vi "20220107_00.vi"() -> ()   [LabVIEW 2019]
uses:
  <vilib>/numeric/Random Number (Range) DBL.vi
panel:
  in  "Flush":bool
  out "enque timed out?":bool
  out "deque timed out?":bool
  out "element":dbl
  in  "Deque":bool
  out "elements":dbl[](array[numeric])
  in  "Lossy Enque":bool
  in  "Enque":bool
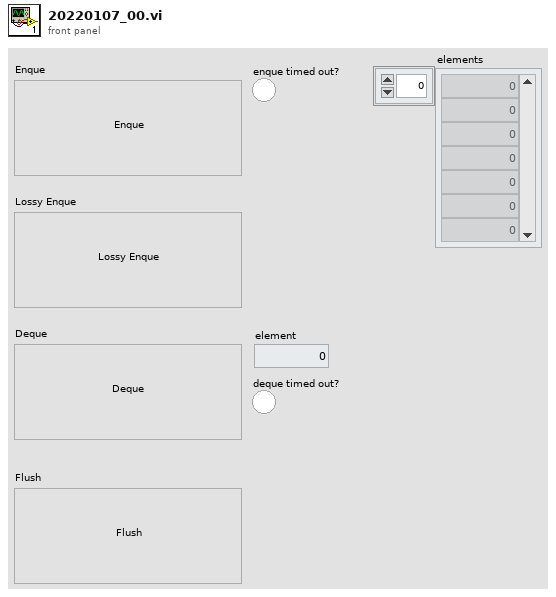
[diagram p1: front panel]
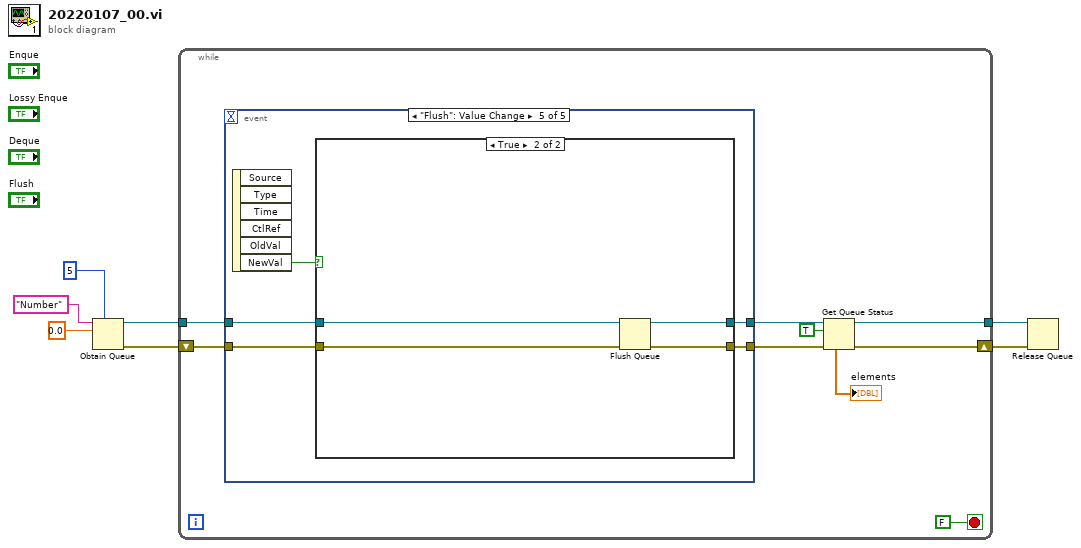
[diagram p0: block diagram]
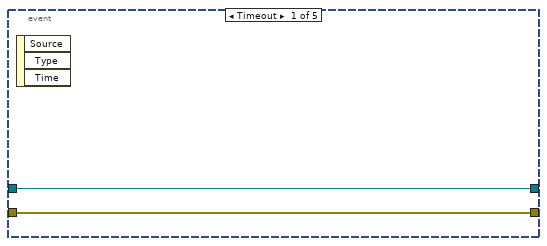
[diagram p2: hidden frame]
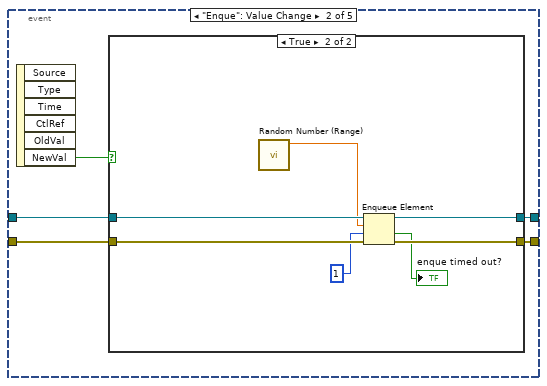
[diagram p3: hidden frame]
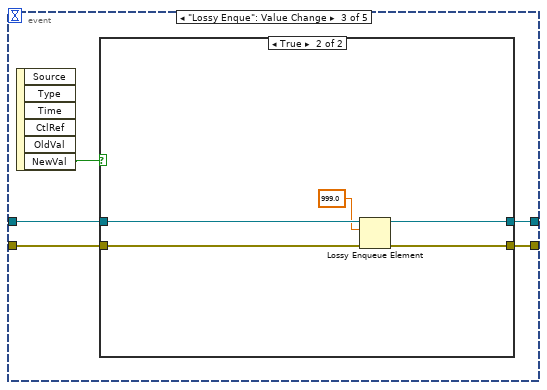
[diagram p5: hidden frame]
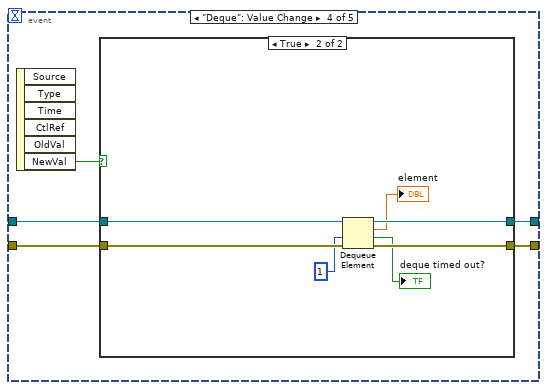
[diagram p7: hidden frame]
diagram:
  n1 = Obtain Queue(max queue size (-1, unlimited)=5, name (unnamed)="Number", element data type=0.0) -> (queue out=w2:refnum<queue>, error out=w3:errorcluster)  [unwired: 2 in, 1 out]
  n2 = while {
    shift-right: [w11] -> w5
    shift-left: w3 -> [w15]
    tunnel: w2 -> [w16]
    tunnel: [w10] -> w4
    stop <- FALSE stop-if-true
    n3 = event shown="[4] \"Flush\": Value Change" {
      selector: _ -> [_ _ _ _ _]
      dyn-events: _ -> [_ _ _ _ _]
      timeout: _ -> [_ _ _ _ _]
      tunnel: w16 -> [w17 w22 w35 w47 w61]
      tunnel: w15 -> [w18 w21 w36 w48 w62]
      tunnel: [w18 w20 w34 w46 w60] -> w13
      tunnel: [w17 w19 w33 w45 w59] -> w12
      event Timeout {
        n4 = event-data() -> ()  [unwired: 1 in, 3 out]
      }
      event "Enque": Value Change {
        n5 = event-data() -> ("NewVal"=w23:bool)  [unwired: 1 in, 5 out]
        n6 = case shown="True" w23 {
          tunnel: w22 -> [w24 w32]
          tunnel: w21 -> [w25 w31]
          tunnel: [w25 w30] -> w20
          tunnel: [w24 w29] -> w19
          frame False {
          }
          frame True {
            n7 = call-poly <vilib>:"Random Number (Range).vi"() -> ("number"=w28:dbl)  [unwired: 11 in]
            n8 = Enqueue Element(queue=w32, element=w28, timeout in ms (-1)=1, error in (no error)=w31) -> (queue out=w29:refnum<queue>, timed out?=→"enque timed out?":bool, error out=w30:errorcluster)
          }
        }
      }
      event "Lossy Enque": Value Change {
        n9 = event-data() -> ("NewVal"=w37:bool)  [unwired: 1 in, 5 out]
        n10 = case shown="True" w37 {
          tunnel: w36 -> [w39 w44]
          tunnel: w35 -> [w38 w43]
          tunnel: [w39 w42] -> w34
          tunnel: [w38 w41] -> w33
          frame False {
          }
          frame True {
            n11 = Lossy Enqueue Element(queue=w43, element=999.0, error in (no error)=w44) -> (queue out=w41:refnum<queue>, error out=w42:errorcluster)  [unwired: 2 out]
          }
        }
      }
      event "Deque": Value Change {
        n12 = event-data() -> ("NewVal"=w49:bool)  [unwired: 1 in, 5 out]
        n13 = case shown="True" w49 {
          tunnel: w48 -> [w51 w58]
          tunnel: w47 -> [w50 w57]
          tunnel: [w51 w56] -> w46
          tunnel: [w50 w55] -> w45
          frame False {
          }
          frame True {
            n14 = Dequeue Element(queue=w57, timeout in ms (-1)=1, error in (no error)=w58) -> (queue out=w55:refnum<queue>, element=→"element":dbl, timed out?=→"deque timed out?":bool, error out=w56:errorcluster)
          }
        }
      }
      event "Flush": Value Change {
        n15 = event-data() -> ("NewVal"=w63:bool)  [unwired: 1 in, 5 out]
        n16 = case shown="True" w63 {
          tunnel: w62 -> [w65 w69]
          tunnel: w61 -> [w64 w66]
          tunnel: [w65 w68] -> w60
          tunnel: [w64 w67] -> w59
          frame False {
          }
          frame True {
            n17 = Flush Queue(queue=w66, error in (no error)=w69) -> (queue out=w67:refnum<queue>, error out=w68:errorcluster)  [unwired: 1 out]
          }
        }
      }
    }
    n18 = Get Queue Status(queue=w12, return elements? (F)=TRUE, error in (no error)=w13) -> (queue out=w10:refnum<queue>, error out=w11:errorcluster, elements=→"elements":dbl[])  [unwired: 5 out]
  }
  n19 = Release Queue(queue=w4, error in (no error)=w5) -> ()  [unwired: 1 in, 3 out]
